vi "Daemon.vi"(6 "Method":enum8{"Back", "Front", "Lossy", "Absent"}(ring), 8 "Message":string, 9 "Time":refnum<data-value>, 10 "Emit":refnum<queue>, 11 "Queue":refnum<queue>) -> ()   [LabVIEW 2021, in "QueueTimer.lvlib"]
doc: "Daemon thread that controls the periodic messaging."
uses:
  QueueTimer.lvlib
  TypeDefs/Timer.ctl
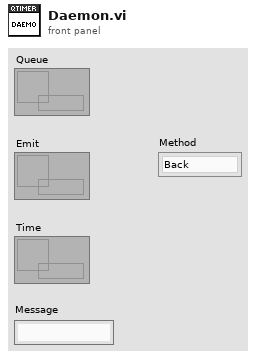
[diagram p1: front panel]
types:
  T1 = typedef "QueueTimer.lvlib/Timer.ctl" = cluster{"Delay":i32, "Start":bool, "Ticks":u32}
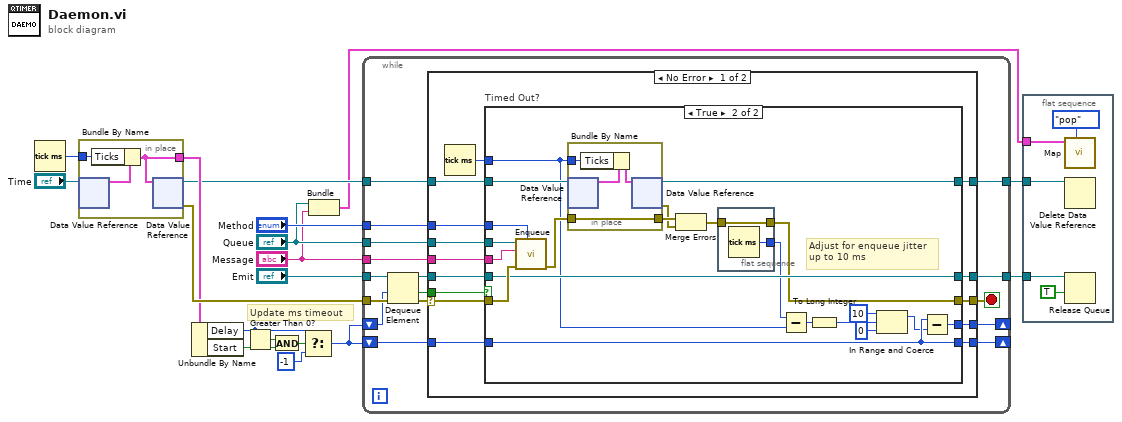
[diagram p0: block diagram]
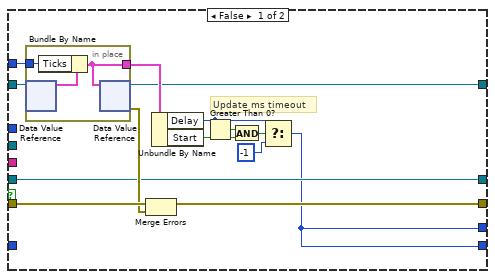
[diagram p2: hidden frame]
diagram:
  # "Update ms timeout"
  n1 = Tick Count (ms)() -> (millisecond timer value=w7:u32)
  n2 = in-place {
    in-place-border: [w20] -> w14
    in-place-border: w7 -> [w19]
    n3 = in-place-dvr #1("Time") -> (w21:T1)  [unwired: 1 out]
    n4 = Bundle By Name(cluster=w21, "Ticks"=w19) -> (w20:T1)
    n5 = in-place-dvr #1(w20) -> (w8:refnum<data-value>, w15:errorcluster)
  }
  n6 = Unbundle By Name(w14) -> ("Delay"=w11:i32, "Start"=w13:bool)
  n7 = Greater Than 0?(x=w11) -> (x > 0?=w9:bool)
  n8 = And(x=w9, y=w13) -> (x .and. y?=w10:bool)
  n9 = Select(t=w11, s=w10, f=-1) -> (s? t:f=w1:i32)
  n10 = Bundle("Queue"="Queue", "Message"="Message") -> (w2:cluster{"Queue":refnum<queue>, "Message":string})  [unwired: 1 in]
  n11 = while {
    tunnel: "Emit" -> [w37]
    shift-right: [w28] -> _
    shift-left: w1 -> [w29]
    tunnel: "Queue" -> [w36]
    tunnel: "Method" -> [w35]
    tunnel: "Message" -> [w34]
    tunnel: w15 -> [w30]
    tunnel: w8 -> [w27]
    tunnel: [w26] -> w6
    tunnel: [w25] -> w5
    shift-right: [w23] -> _
    shift-left: w1 -> [w22]
    stop <- w32 stop-if-true
    n12 = Dequeue Element(queue=w37, timeout in ms (-1)=w22, error in (no error)=w30) -> (queue out=w24:refnum<queue>, timed out?=w31:bool, error out=w33:errorcluster)  [unwired: 1 out]
    n13 = case shown="No Error" w33 {
      selector: w33 -> [w48 w99]
      tunnel: w36 -> [w51 _]
      tunnel: w35 -> [w50 _]
      tunnel: w34 -> [w49 _]
      tunnel: [w47 w99] -> w32
      tunnel: w31 -> [w46 _]
      tunnel: w29 -> [w42 w96]
      tunnel: [w43 w96] -> w28
      tunnel: w27 -> [w44 w98]
      tunnel: [w41 w98] -> w26
      tunnel: [w40 w97] -> w25
      tunnel: w24 -> [w39 w97]
      tunnel: [w38 w96] -> w23
      frame No Error {
        n14 = Tick Count (ms)() -> (millisecond timer value=w45:u32)
        n15 = case "Timed Out?" shown="True" w46 {
          tunnel: w51 -> [_ w89]
          tunnel: w50 -> [_ w88]
          tunnel: w49 -> [_ w87]
          tunnel: w48 -> [w65 w86]
          tunnel: [w59 w78] -> w47
          tunnel: w45 -> [w57 w76]
          tunnel: w44 -> [w58 w85]
          tunnel: [w52 w75] -> w43
          tunnel: w42 -> [_ w75]
          tunnel: [w54 w81] -> w41
          tunnel: [w53 w80] -> w40
          tunnel: w39 -> [w53 w80]
          tunnel: [w52 w73] -> w38
          frame False {
            # "Update ms timeout"
            n16 = in-place {
              in-place-border: [w67] -> w56
              in-place-border: w57 -> [w66]
              n17 = in-place-dvr #2(w58) -> (w68:T1)  [unwired: 1 out]
              n18 = Bundle By Name(cluster=w68, "Ticks"=w66) -> (w67:T1)
              n19 = in-place-dvr #2(w67) -> (w54:refnum<data-value>, w55:errorcluster)
            }
            n20 = Merge Errors(w65, w55) -> (w59:errorcluster)
            n21 = Unbundle By Name(w56) -> ("Delay"=w62:i32, "Start"=w60:bool)
            n22 = Greater Than 0?(x=w62) -> (x > 0?=w64:bool)
            n23 = And(x=w64, y=w60) -> (x .and. y?=w63:bool)
            n24 = Select(t=w62, s=w63, f=-1) -> (s? t:f=w52:i32)
          }
          frame True {
            # "Adjust for enqueue jitter\nup to 10 ms"
            n25 = call "Enqueue.vi"("Method (Back)"=w88, "error in (no error)"=w86, "Element"=w87, "Queue in"=w89) -> ("error out"=w83:errorcluster)  [unwired: 6 in, 1 out]
            n26 = in-place {
              in-place-border: w76 -> [w93]
              in-place-border: [w92] -> w84
              in-place-border: w83 -> [w92]
              n27 = in-place-dvr #3(w85) -> (w95:T1)  [unwired: 1 out]
              n28 = Bundle By Name(cluster=w95, "Ticks"=w93) -> (w94:T1)
              n29 = in-place-dvr #3(w94) -> (w81:refnum<data-value>, w82:errorcluster)
            }
            n30 = Merge Errors(w84, w82) -> (w79:errorcluster)
            n31 = flat-sequence {
              tunnel: [w91] -> w78
              tunnel: w79 -> [w91]
              tunnel: [w90] -> w77
              frame #0 {
                n32 = Tick Count (ms)() -> (millisecond timer value=w90:u32)
              }
            }
            n33 = Subtract(x=w77, y=w76) -> (x-y=w74:u32)
            n34 = To Long Integer(number=w74) -> (32bit integer=w72:i32)
            n35 = In Range and Coerce(upper limit=10, x=w72, lower limit=0) -> (coerced(x)=w71:i32)  [unwired: 1 out]
            n36 = Subtract(x=w75, y=w71) -> (x-y=w73:i32)
          }
        }
      }
      frame Error {
      }
    }
  }
  n37 = flat-sequence {
    tunnel: w6 -> [w104]
    tunnel: w5 -> [w103]
    tunnel: w2 -> [w100]
    frame #0 {
      n38 = call "Map.vi"("Action"=enum8{"noop", "get", "set", "pop"}."pop", "Timer Id"=w100) -> ()  [unwired: 7 in, 3 out]
      n39 = Delete Data Value Reference(data value reference=w104) -> ()  [unwired: 1 in, 2 out]
      n40 = Release Queue(queue=w103, force destroy? (F)=TRUE) -> ()  [unwired: 1 in, 3 out]
    }
  }
